vi "GetAllCtrls.vi"(1 "Prefix":string, 2 "VI":refnum<vi>) -> (0 "Ctrls":cluster{"Name":string, "Ctrl":refnum<vi>}[](array[cluster]))   [LabVIEW 2014]
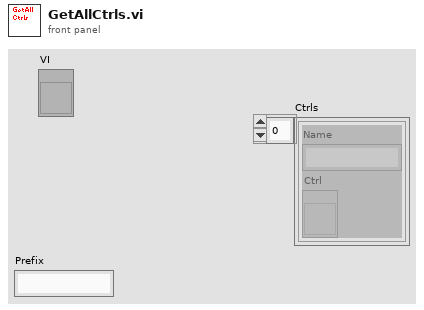
[diagram p1: front panel]
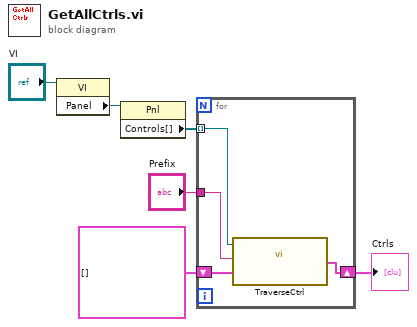
[diagram p0: block diagram]
diagram:
  n1 = property class="VI"(reference="VI") -> ("Panel"=w6:refnum<vi>)  [unwired: 1 in, 2 out]
  n2 = property class="Pnl"(reference=w6) -> ("Controls[]"=w5:refnum<vi>[])  [unwired: 1 in, 2 out]
  n3 = for {
    tunnel: w5 -> [w10] mode=indexing
    shift-right: [w9] -> w2
    shift-left: cluster{"Name":string, "Ctrl":refnum<vi>}[] [] ("Array") -> [w7]
    tunnel: "Prefix" -> [w8]
    n4 = call "TraverseCtrl.vi"("Input"=w7, "Prefix"=w8, "Ctrl Reference"=w10) -> ("Output"=w9:cluster{"Name":string, "Ctrl":refnum<vi>}[])
  }
  "Ctrls" <- w2
